vi "remove_outside_pairs_on_inside_pairs.vi"(9 "Inside Pair Offset":cluster{"Start Offset":i32, "End offset":i32}[](array[cluster]), 10 "Outside Pair Offset":cluster{"Start Offset":i32, "End offset":i32}[](array[cluster]), 11 "Instrument Command In":string) -> (3 "Instrument Command Out":string)   [LabVIEW 2018]
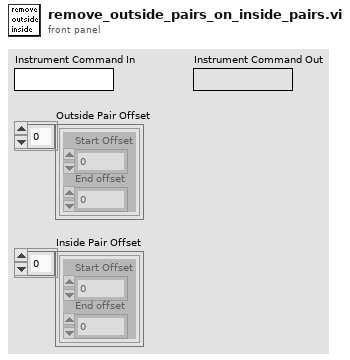
[diagram p1: front panel]
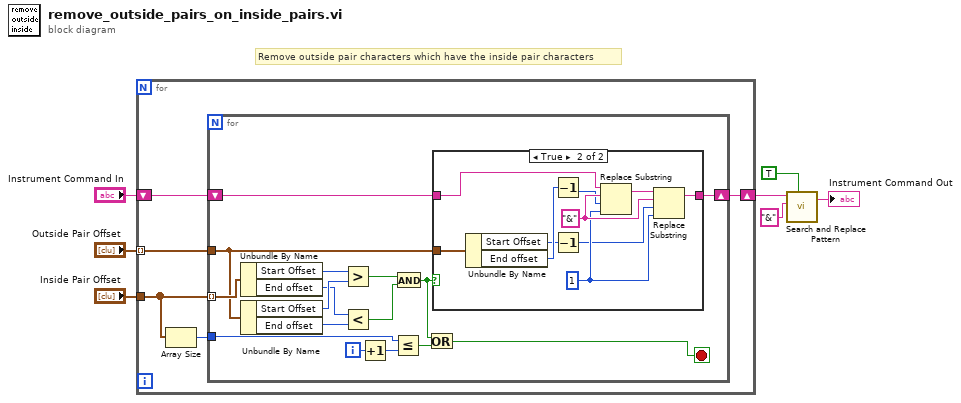
[diagram p0: block diagram]
diagram:
  # "Remove outside pair characters which have the inside pair characters"
  n1 = for {
    tunnel: "Outside Pair Offset" -> [w12] mode=indexing
    tunnel: "Inside Pair Offset" -> [w11]
    shift-right: [w8] -> w6
    shift-left: "Instrument Command In" -> [w9]
    n2 = Array Size(array=w11) -> (size(s)=w10:i32)
    n3 = for {
      tunnel: w11 -> [w28] mode=indexing
      tunnel: w12 -> [w21]
      tunnel: w10 -> [w18]
      shift-right: [w14] -> w8
      shift-left: w9 -> [w15]
      i -> [w19]
      stop <- w13 stop-if-true
      n4 = Unbundle By Name(w28) -> ("Start Offset"=w27:i32, "End offset"=w25:i32)
      n5 = Unbundle By Name(w21) -> ("Start Offset"=w26:i32, "End offset"=w24:i32)
      n6 = Greater?(x=w27, y=w26) -> (0:w23:bool)
      n7 = Less?(x=w25, y=w24) -> (x < y?=w22:bool)
      n8 = Increment(x=w19) -> (x+1=w16:i32)
      n9 = Less Or Equal?(x=w18, y=w16) -> (x <= y?=w17:bool)
      n10 = And(x=w23, y=w22) -> (x .and. y?=w20:bool)
      n11 = Or(x=w20, y=w17) -> (x .or. y?=w13:bool)
      n12 = case shown="True" w20 {
        tunnel: w21 -> [_ w39]
        tunnel: w15 -> [w29 w35]
        tunnel: [w29 w34] -> w14
        frame False {
        }
        frame True {
          w37 = "&" ("substring (\"\")")
          w36 = 1 ("length (len. of substring)")
          n13 = Unbundle By Name(w39) -> ("Start Offset"=w32:i32, "End offset"=w33:i32)
          n14 = Decrement(x=w33) -> (x-1=w30:i32)
          n15 = Decrement(x=w32) -> (x-1=w31:i32)
          n16 = Replace Substring(2:w36, 3:w30, 4:w37, 5:w35) -> (1:w38:string)  [unwired: 1 out]
          n17 = Replace Substring(2:w36, 3:w31, 4:w37, 5:w38) -> (1:w34:string)  [unwired: 1 out]
        }
      }
    }
  }
  n18 = call <vilib>:"Search and Replace Pattern.vi"("string"=w6, "regular expression (\"\")"="&" ("regular expression (\"\")"), "replace all? (F)"=TRUE) -> ("result string"=→"Instrument Command Out":string)  [unwired: 1 in, 2 out]
